vi "Motor Visa.vi"(8 "错误输入（无错误）":errorcluster, 10 "Command":string, 11 "VISA资源名称":refnum<visa-resource-name>) -> (0 "错误输出":errorcluster, 2 "读取缓冲区":string, 3 "VISA资源名称输出":refnum<visa-resource-name>)   [LabVIEW 2017]
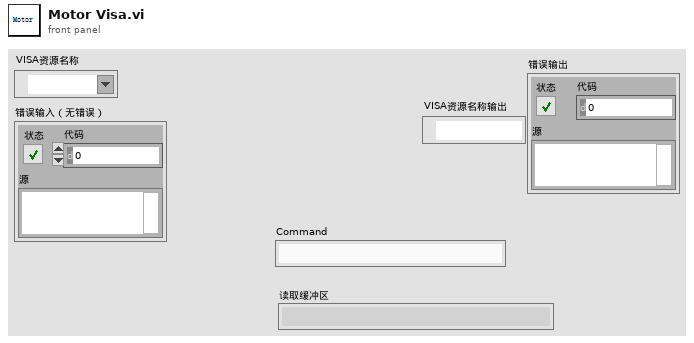
[diagram p1: front panel]
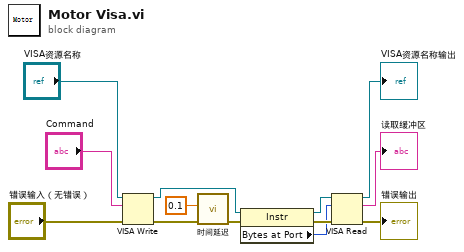
[diagram p0: block diagram]
diagram:
  n1 = VISA Write(VISA resource name="VISA资源名称", write buffer="Command", error in (no error)="错误输入（无错误）") -> (VISA resource name out=w11:refnum<visa-resource-name>, error out=w12:errorcluster)  [unwired: 1 out]
  n2 = call "时间延迟"("error in (no error)"=w12, "Delay Time (s)"=0.1) -> ("error out"=w10:errorcluster)  [unwired: 9 in]
  n3 = property class="Instr"(reference=w11, error in=w10) -> (reference out=w9:refnum<visa-resource-name>, error out=w8:errorcluster, "Bytes at Port"=w7:u32)
  n4 = VISA Read(VISA resource name=w9, byte count=w7, error in (no error)=w8) -> (VISA resource name out=→"VISA资源名称输出":refnum<visa-resource-name>, read buffer=→"读取缓冲区":string, error out=→"错误输出":errorcluster)  [unwired: 1 out]
